vi "Monitor for NTCP Close.vi"(6 "Skip":T1, 7 "timeout":i32=200, 8 "error in (no error)":errorcluster, 9 "From NTCP In":refnum<queue>, 11 "MM Button Events In":refnum<notifier>) -> (0 "error out":errorcluster, 1 "From NTCP Out":refnum<queue>, 2 "Close Received":bool, 3 "Button Events Out":refnum<notifier>)   [LabVIEW 2009]
uses:
  Mixed Mode Button Events Message.ctl
  Mixed Mode Button Events.ctl
  Mixed Mode Widget Button States.ctl
  NTCP Client/NTCP 2 MM Message.ctl
  NTCP library/NTCP Commands.ctl
  Target.ctl
  Data Access Objects/Metadata/LBCB Number.ctl
  Skip NTCP Close Monitor.ctl
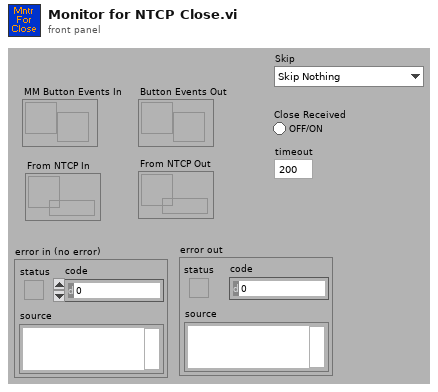
[diagram p1: front panel]
types:
  T1 = typedef "Skip NTCP Close Monitor.ctl" = enum16{"Skip Nothing", "Skip NTCP", "Skip Button Event"}
  T2 = typedef "NTCP 2 MM Message.ctl" = cluster{"NTCP commands":T3, "Transaction ID":string, "Control Point":string, "Targets":T4[]}
  T3 = typedef "NTCP Commands.ctl" = enum16{"propose", "execute", "cancel", "set-parameter", "get-parameter", "open-session", "close-session", "get-control-point", "Unknown", "stop"}
  T4 = typedef "Target.ctl" = cluster{"LBCB Number":T5, "DOF Vectors":enum16{" ", "Dx", "Dy", "Dz", "Rx", "Ry", "Rz", "Fx", "Fy", "Fz", "Mx", "My", "Mz"}, "Amount":dbl}
  T5 = typedef "LBCB Number.ctl" = enum16{"LBCB1", "LBCB2"}
  T6 = typedef "Mixed Mode Button Events Message.ctl" = cluster{"MM Control Events":T7, "Button States":T8}
  T7 = typedef "Mixed Mode Button Events.ctl" = enum16{"Propose.Accept", "Propose.Decline", "Execute.Start", "Execute.Stop", "TargetSet", "InputFile.Load", "InputFile.Reset", "InputFile.Pause", "InputFile.Run", "CartesianType.Changed", "NCTP.ConnectToServer", "Application.Stop", "Control.Enabled", "Control.Disabled", "ControlType.Changed", "Nop"}
  T8 = typedef "Mixed Mode Widget Button States.ctl" = cluster{"Auto-Start Enabled":bool, "Auto-Accept Enabled":bool, "Exit Requested":bool, "Input File Loaded":bool, "Input File Running":bool, "NTCP Server  On":bool}
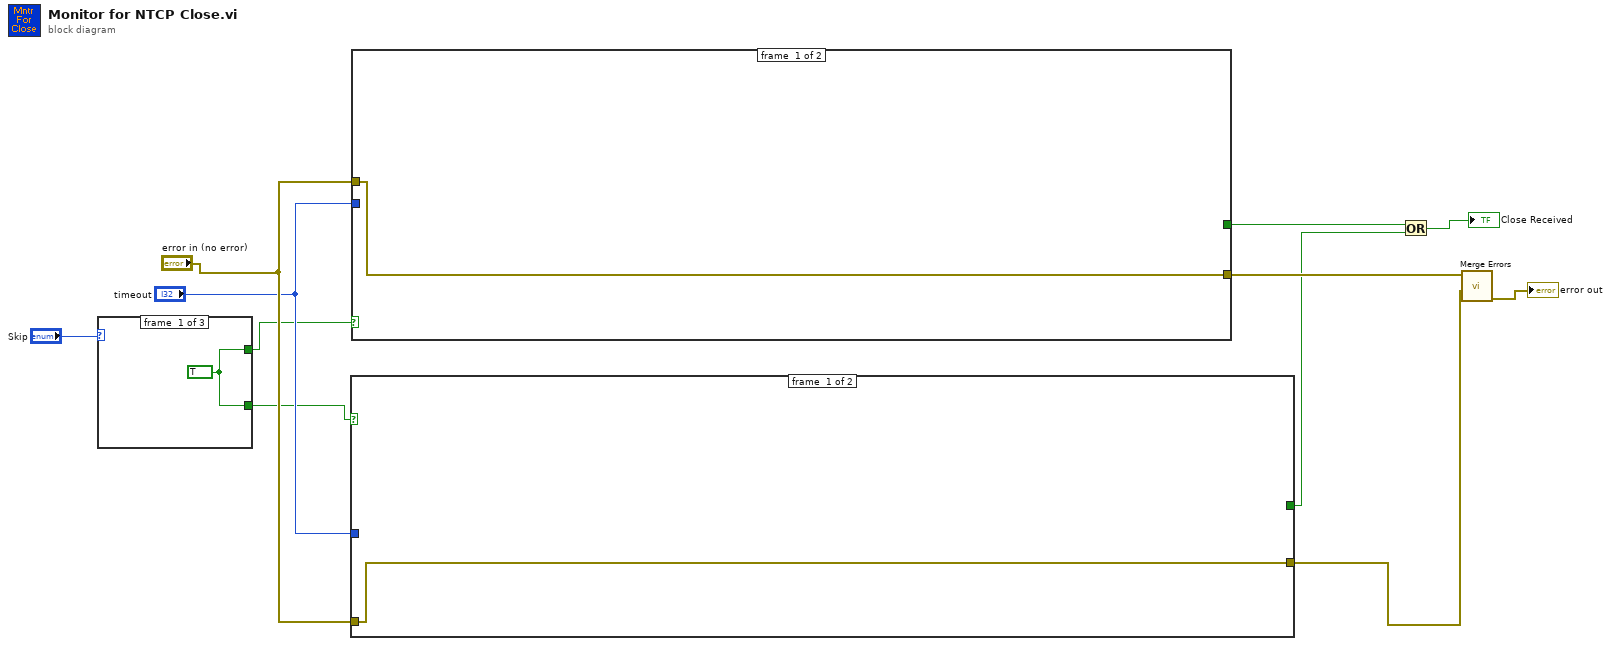
[diagram p0: block diagram]
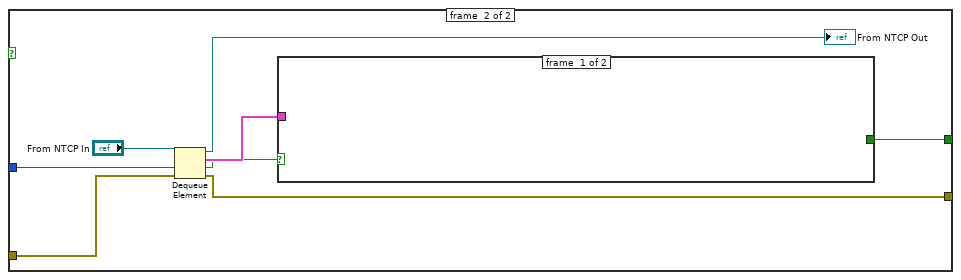
[diagram p2: hidden frame]
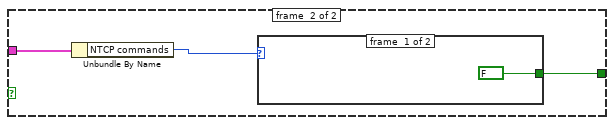
[diagram p3: hidden frame]
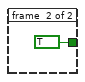
[diagram p4: hidden frame]
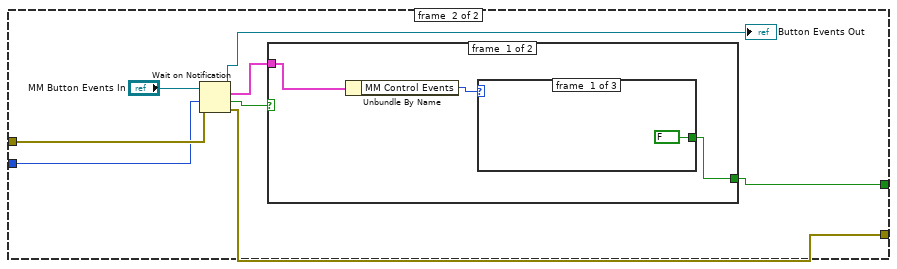
[diagram p5: hidden frame]
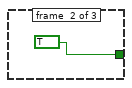
[diagram p6: hidden frame]
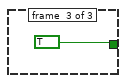
[diagram p7: hidden frame]
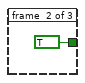
[diagram p9: hidden frame]
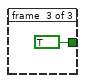
[diagram p10: hidden frame]
diagram:
  n1 = case shown="\"Skip NTCP\"" "Skip" {
    tunnel: [w12 TRUE _] -> w2
    tunnel: [w12 _ TRUE] -> w1
    frame #0 {
      w12 = TRUE
    }
    frame #1 {
    }
    frame #2 {
    }
  }
  n2 = case shown="True" w1 {
    tunnel: "error in (no error)" -> [w15 w20]
    tunnel: "timeout" -> [_ w19]
    tunnel: [w15 w17] -> w4
    tunnel: [_ w16] -> w3
    frame #0 {
    }
    frame #1 {
      n3 = Dequeue Element(queue="From NTCP In", timeout in ms (-1)=w19, error in (no error)=w20) -> (queue out=→"From NTCP Out":refnum<queue>, element=w23:T2, timed out?=w22:bool, error out=w17:errorcluster)
      n4 = case shown="True" w22 {
        tunnel: w23 -> [_ w26]
        tunnel: [_ w24] -> w16
        frame #0 {
        }
        frame #1 {
          n5 = Unbundle By Name(w26) -> ("NTCP commands"=w25:T3)
          n6 = case shown="\"close-session\"" w25 {
            tunnel: [FALSE TRUE] -> w24
            frame #0 {
            }
            frame #1 {
            }
          }
        }
      }
    }
  }
  n7 = case shown="True" w2 {
    tunnel: [_ w33] -> w10
    tunnel: [w29 w32] -> w7
    tunnel: "error in (no error)" -> [w29 w31]
    tunnel: "timeout" -> [_ w30]
    frame #0 {
    }
    frame #1 {
      n8 = Wait on Notification(notifier="MM Button Events In", timeout in ms (-1)=w30, error in (no error)=w31) -> (notifier out=→"Button Events Out":refnum<notifier>, notification=w34:T6, timed out?=w35:bool, error out=w32:errorcluster)  [unwired: 1 in]
      n9 = case shown="False" w35 {
        tunnel: w34 -> [w40 _]
        tunnel: [w38 _] -> w33
        frame #0 {
          n10 = Unbundle By Name(w40) -> ("MM Control Events"=w39:T7)
          n11 = case shown="\"Execute.Start\", Default" w39 {
            tunnel: [FALSE TRUE TRUE] -> w38
            frame #0 {
            }
            frame #1 {
            }
            frame #2 {
            }
          }
        }
        frame #1 {
        }
      }
    }
  }
  n12 = Or(x=w10, y=w3) -> (x .or. y?=→"Close Received":bool)
  n13 = call <vilib>:"Merge Errors.vi"("error in 3 (no error)"=w4, "error in 1 (no error)"=w7) -> ("error out"=→"error out":errorcluster)  [unwired: 5 in]
